vi "DSC Device and User Paths.vi"(7 "instrument":T1) -> (2 "User Path":refnum<k21>, 3 "Device Path":refnum<k21>)   [LabVIEW 2016, in "Control Experiment.lvclass"]
uses:
  Control Experiment.lvclass
  Typedefs/Instrument--enum.ctl
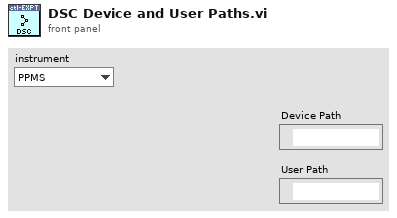
[diagram p1: front panel]
types:
  T1 = typedef "Control Experiment.lvclass/Instrument--enum.ctl" = enum16{"PPMS", "PPMS2", "DR200", "MNK", "CF900", "MFP3D", "CYPHER", "AGILENT", "JEOL", "THz1", "THz2", "EBL"}
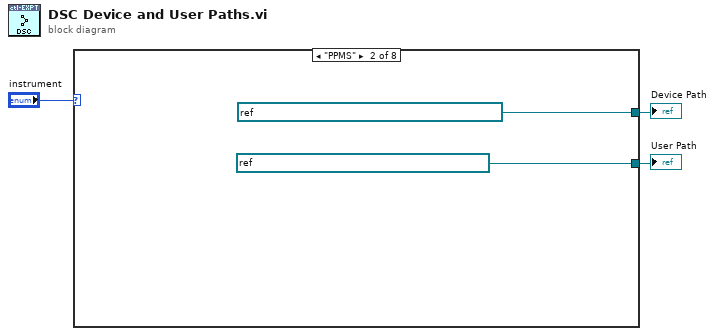
[diagram p0: block diagram]
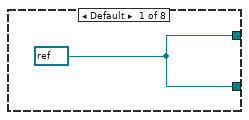
[diagram p2: hidden frame]
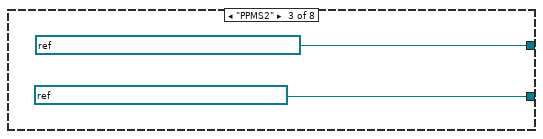
[diagram p3: hidden frame]
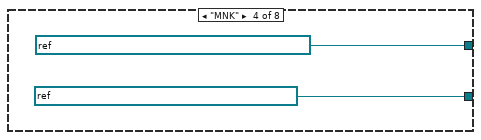
[diagram p4: hidden frame]
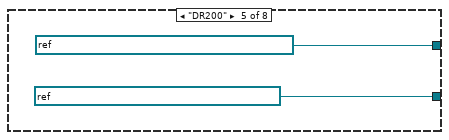
[diagram p5: hidden frame]
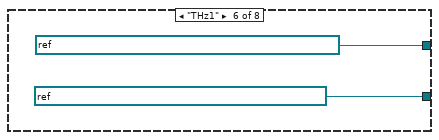
[diagram p6: hidden frame]
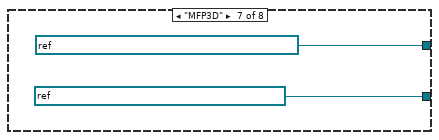
[diagram p7: hidden frame]
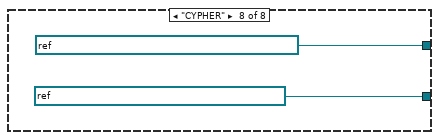
[diagram p8: hidden frame]
diagram:
  n1 = case shown="\"PPMS\"" "instrument" {
    tunnel: [w4 refnum<k21> "ni.var.psp://housesoftheholy/PPMS 1/Device" ("Device Path") refnum<k21> "ni.var.psp://housesoftheholy/PPMS 2/Device" ("Device Path") refnum<k21> "ni.var.psp://housesoftheholy/MNK_18T/Device" ("Device Path") refnum<k21> "ni.var.psp://housesoftheholy/DR200/Device" ("Device Path") refnum<k21> "ni.var.psp://housesoftheholy/Montana THZ1/Device" ("Device Path") refnum<k21> "ni.var.psp://housesoftheholy/MFP3D/Device" ("Device Path") refnum<k21> "ni.var.psp://housesoftheholy/Cypher/Device" ("Device Path")] -> w2
    tunnel: [w4 refnum<k21> "ni.var.psp://housesoftheholy/PPMS 1/User" ("Device Path") refnum<k21> "ni.var.psp://housesoftheholy/PPMS 2/User" ("Device Path") refnum<k21> "ni.var.psp://housesoftheholy/MNK_18T/User" ("Device Path") refnum<k21> "ni.var.psp://housesoftheholy/DR200/User" ("Device Path") refnum<k21> "ni.var.psp://housesoftheholy/Montana THZ1/User" ("Device Path") refnum<k21> "ni.var.psp://housesoftheholy/MFP3D/User" ("Device Path") refnum<k21> "ni.var.psp://housesoftheholy/Cypher/User" ("Device Path")] -> w1
    frame Default {
      w4 = refnum<k21> refnum ("Device Path")
    }
    frame "PPMS" {
    }
    frame "PPMS2" {
    }
    frame "MNK" {
    }
    frame "DR200" {
    }
    frame "THz1" {
    }
    frame "MFP3D" {
    }
    frame "CYPHER" {
    }
  }
  "Device Path" <- w2
  "User Path" <- w1
